vi "Globals.vi"() -> ()   [LabVIEW 2025]
panel:
  in  "Flywheel Ready?":bool
  in  "Pivot Out?":bool
  in  "Game Data":string
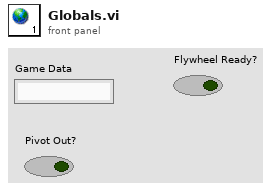
[diagram p1: front panel]
diagram:
